vi "Drivebase Immediate Wrapper.vi"() -> ()   [LabVIEW 2019]
uses:
  Implementation/Drive Base Operations.ctl
panel:
  in  "Right Setpoint":dbl
  in  "Left Setpoint":dbl
  in  "Operation":T1
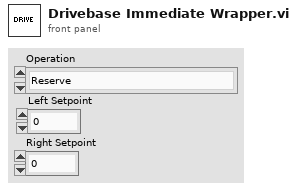
[diagram p1: front panel]
types:
  T1 = typedef "Drive Base Operations.ctl" = enum16{"Reserve", "Read Current", "Immediate", "Immediate Limelight", "Immediate Duration", "Limelight", "Manual Adjustment", "Play Path"}
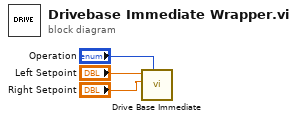
[diagram p0: block diagram]
diagram:
  n1 = call "Drive Base Immediate.vi"("Operation"="Operation", "Right Setpoint"="Right Setpoint", "Left Setpoint"="Left Setpoint") -> ()  [unwired: 8 in, 1 out]
